vi "Variant_AppendElementToCluster.vi"(7 "Path":string, 9 "Element name":string, 10 "Element":variant, 11 "Data in":variant) -> (3 "Data out":variant)   [LabVIEW 2013, in "OpenVariant.lvlib"]
uses:
  OpenVariant.lvlib
  TypeDescriptor/OpenDescriptor.lvlib
  Conversions/OpenConvert.lvlib
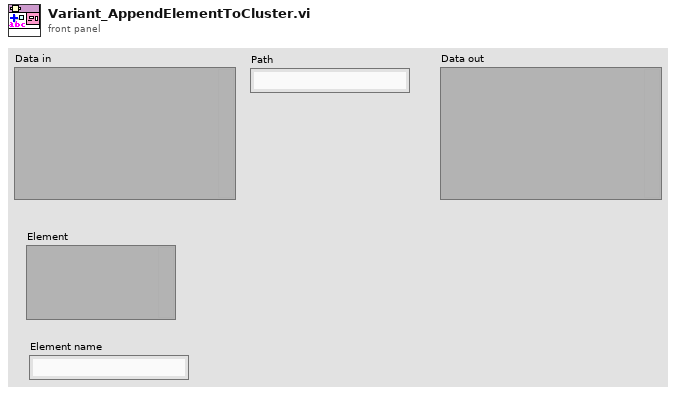
[diagram p1: front panel]
types:
  T1 = typedef "OpenDescriptor.lvlib/Descriptor Element -- cluster.ctl" = cluster{"type descriptor":i16[], "name":string, "class":string, "data string":string}
  T2 = typedef "Type Descriptor I16 Array.ctl" = T3[]
  T3 = typedef "Type Descriptor I16.ctl" = i16
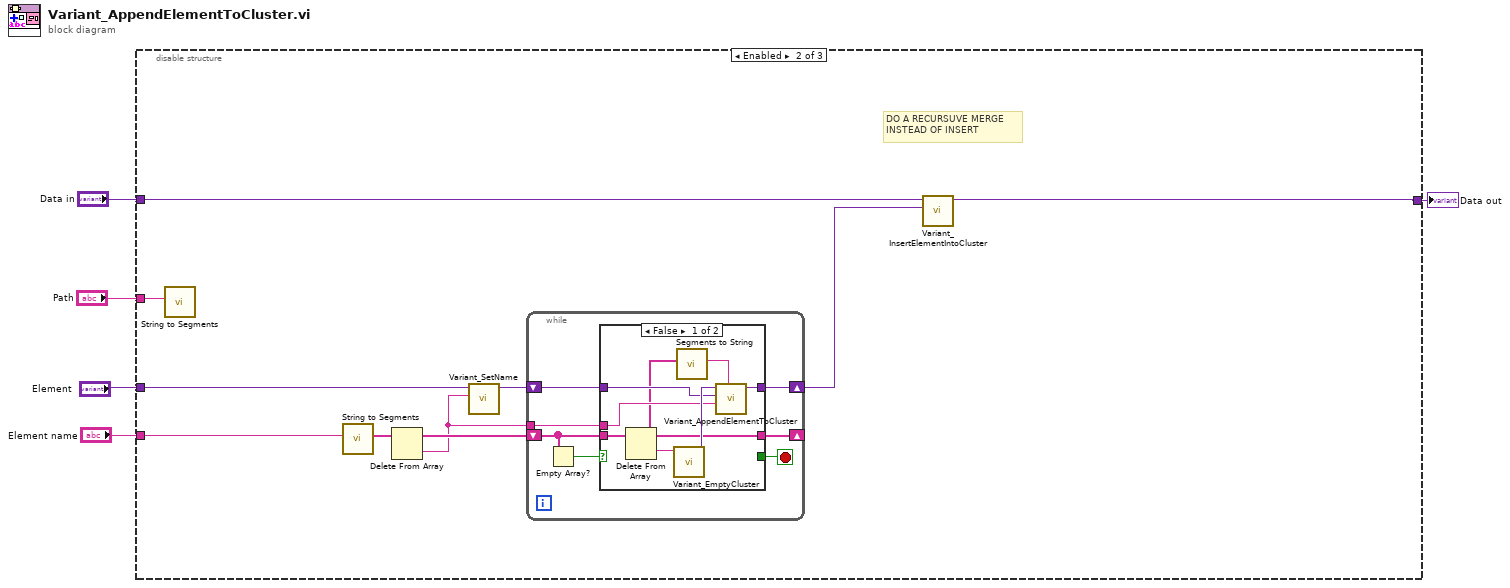
[diagram p0: block diagram]
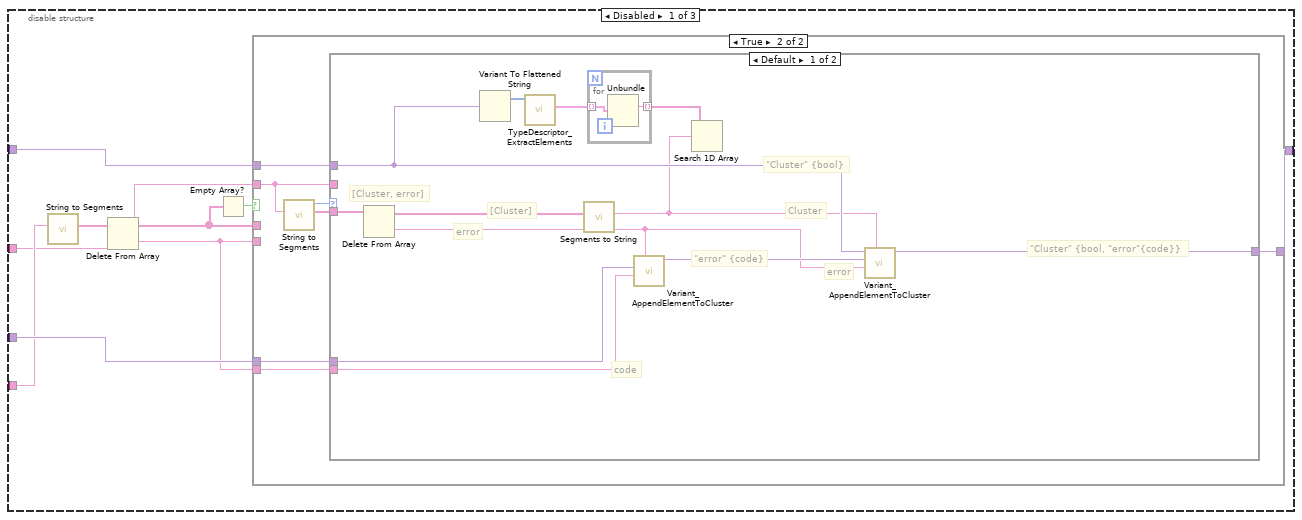
[diagram p2: hidden frame]
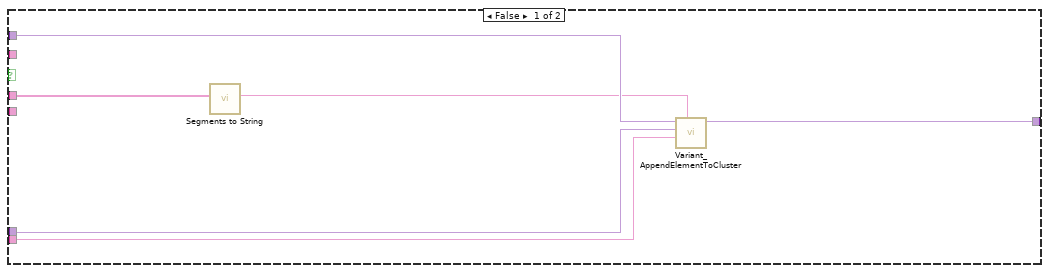
[diagram p3: hidden frame]
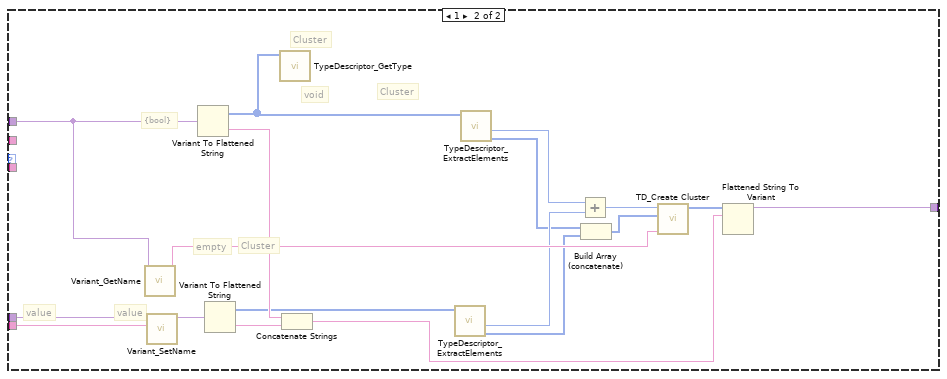
[diagram p4: hidden frame]
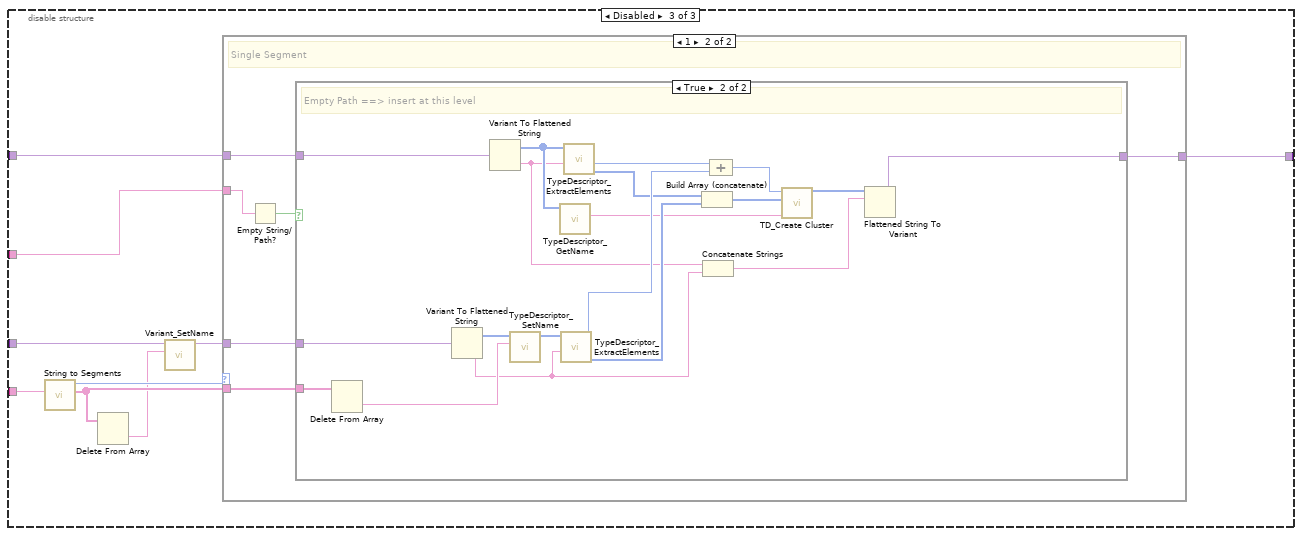
[diagram p6: hidden frame]
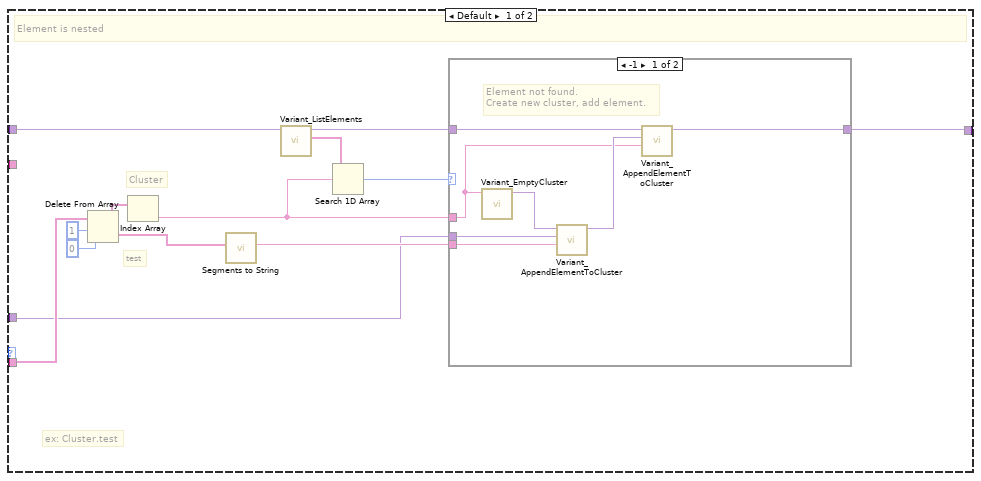
[diagram p7: hidden frame]
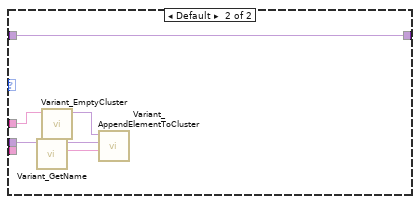
[diagram p8: hidden frame]
diagram:
  n1 = disable-structure shown="Enabled" {
    disable-tunnel: "Element" -> [w14 w67 w90]
    disable-tunnel: [w13 w62 w92] -> w4
    disable-tunnel: "Data in" -> [w12 w64 w94]
    disable-tunnel: "Element name" -> [w8 w69 w96]
    disable-tunnel: "Path" -> [w6 w60 w93]
    frame Disabled {
      n2 = call "String to Segments.vi"("String"=w8) -> ("Segments"=w11:string[])  [unwired: 9 in, 1 out]
      n3 = Delete From Array(array=w11) -> (deleted portion=w7:string, array with subset deleted=w10:string[])  [unwired: 2 in]
      n4 = Empty Array?(array=w10) -> (empty?=w9:bool)
      n5 = case shown="True" w9 {
        tunnel: w7 -> [w18 w27]
        tunnel: w14 -> [w19 w26]
        tunnel: [w20 w25] -> w13
        tunnel: w12 -> [w17 w24]
        tunnel: w7 -> [_ _]
        tunnel: w10 -> [w16 _]
        tunnel: w6 -> [_ w23]
        frame False {
          n6 = call "Segments to String.vi"("Segments"=w16) -> ("String"=w15:string)  [unwired: 10 in]
          n7 = call "Variant_AppendElementToCluster.vi"("Path"=w15, "Element name"=w18, "Element"=w19, "Data in"=w17) -> ("Data out"=w20:variant)  [unwired: 7 in]
        }
        frame True {
          n8 = call "String to Segments.vi"("String"=w23) -> ("Segments"=w21:string[], "Nb segments"=w22:i32)  [unwired: 9 in]
          n9 = case shown="Default" w22 {
            tunnel: w27 -> [w39 w57]
            tunnel: w26 -> [w38 w56]
            tunnel: [w34 w54] -> w25
            tunnel: w24 -> [w29 w52]
            tunnel: w23 -> [_ _]
            tunnel: w21 -> [w37 _]
            frame Default {
              # "\"Cluster\" {bool, \"error\"{code}}"
              # "error"
              # "\"error\" {code}"
              # "\"Cluster\" {bool}"
              # "code"
              # "error"
              # "Cluster"
              # "[Cluster]"
              # "[Cluster, error]"
              n10 = Delete From Array(array=w37) -> (deleted portion=w33:string, array with subset deleted=w36:string[])  [unwired: 2 in]
              n11 = Variant To Flattened String(Variant=w29) -> (1:w30:i16[])  [unwired: 1 out]
              n12 = call "TypeDescriptor_ExtractElements.vi"("type descriptor"=w30) -> ("elements"=w31:T1[])  [unwired: 7 in, 3 out]
              n13 = call "Segments to String.vi"("Segments"=w36) -> ("String"=w28:string)  [unwired: 10 in]
              n14 = for {
                tunnel: w31 -> [w41] mode=indexing
                tunnel: [w40] -> w32 mode=indexing
                n15 = Unbundle(w41) -> ("name"=w40:string)  [unwired: 3 out]
              }
              n16 = call "Variant_AppendElementToCluster.vi"("Path"=w33, "Element name"=w39, "Element"=w38) -> ("Data out"=w35:variant)  [unwired: 8 in]
              n17 = Search 1D Array(1D array=w32, element=w28) -> ()  [unwired: 1 in, 1 out]
              n18 = call "Variant_AppendElementToCluster.vi"("Path"=w28, "Element name"=w33, "Element"=w35, "Data in"=w29) -> ("Data out"=w34:variant)  [unwired: 7 in]
            }
            frame 1 {
              # "Cluster"
              # "Cluster"
              # "Cluster"
              # "{bool}"
              # "value"
              # "value"
              # "empty"
              # "void"
              n19 = call "Variant_GetName.vi"("Variant"=w52) -> ("Name"=w51:string)  [unwired: 8 in, 2 out]
              n20 = call "Variant_SetName.vi"("Name"=w57, "Variant"=w56) -> ("Named Variant"=w55:variant)  [unwired: 9 in]
              n21 = Variant To Flattened String(Variant=w52) -> (data string=w59:string, 1:w50:i16[])
              n22 = Variant To Flattened String(Variant=w55) -> (data string=w49:string, 1:w58:i16[])
              n23 = call "TypeDescriptor_GetType.vi"("type descriptor"=w50) -> ()  [unwired: 9 in, 2 out]
              n24 = Concatenate Strings(w59, w49) -> (w53:string)
              n25 = call "TypeDescriptor_ExtractElements.vi"("type descriptor"=w58) -> ("concatenated element descriptors"=w44:i16[], "Nb elements"=w45:i32)  [unwired: 7 in, 2 out]
              n26 = call "TypeDescriptor_ExtractElements.vi"("type descriptor"=w50) -> ("concatenated element descriptors"=w42:i16[], "Nb elements"=w43:i32)  [unwired: 7 in, 2 out]
              n27 = Add(x=w43, y=w45) -> (x+y=w46:i32)
              n28 = Build Array (concatenate)(w42, w44) -> (w48:i16[])
              n29 = call <vilib>:"TD_Create Cluster.vi"("Name"=w51, "Concatenated Elts"=w48, "N Elts"=w46) -> ("ClusterTD"=w47:T2)  [unwired: 8 in]
              n30 = Flattened String To Variant(6:w53, 7:w47) -> (3:w54:variant)  [unwired: 1 in, 1 out]
            }
          }
        }
      }
    }
    frame Enabled {
      # "DO A RECURSUVE MERGE\nINSTEAD OF INSERT"
      n31 = call "String to Segments.vi"("String"=w60) -> ()  [unwired: 9 in, 2 out]
      n32 = call "String to Segments.vi"("String"=w69) -> ("Segments"=w68:string[])  [unwired: 9 in, 1 out]
      n33 = Delete From Array(array=w68) -> (deleted portion=w61:string, array with subset deleted=w66:string[])  [unwired: 2 in]
      n34 = call "Variant_SetName.vi"("Name"=w61, "Variant"=w67) -> ("Named Variant"=w65:variant)  [unwired: 9 in]
      n35 = while {
        shift-right: [w74] -> _
        shift-left: w66 -> [w73]
        shift-right: [w71] -> w63
        shift-left: w65 -> [w72]
        tunnel: w61 -> [w70]
        stop <- w75 stop-if-true
        n36 = Empty Array?(array=w73) -> (empty?=w76:bool)
        n37 = case shown="False" w76 {
          selector: w76 -> [_ w87]
          tunnel: [_ w87] -> w75
          tunnel: [w78 w86] -> w74
          tunnel: w73 -> [w84 w86]
          tunnel: w72 -> [w82 w85]
          tunnel: [w81 w85] -> w71
          tunnel: w70 -> [w79 _]
          frame False {
            n38 = Delete From Array(array=w84) -> (deleted portion=w80:string, array with subset deleted=w78:string[])  [unwired: 2 in]
            n39 = call "Variant_EmptyCluster.vi"("Cluster Name"=w80) -> ("Empty Cluster"=w83:variant)  [unwired: 10 in]
            n40 = call "Segments to String.vi"("Segments"=w78) -> ("String"=w77:string)  [unwired: 10 in]
            n41 = call "Variant_AppendElementToCluster.vi"("Path"=w77, "Element name"=w79, "Element"=w82, "Data in"=w83) -> ("Data out"=w81:variant)  [unwired: 7 in]
          }
          frame True {
          }
        }
      }
      n42 = call "Variant_InsertElementIntoCluster.vi"("Element"=w63, "Cluster in"=w64) -> ("Cluster out"=w62:variant)  [unwired: 9 in]
    }
    frame Disabled {
      n43 = call "String to Segments.vi"("String"=w96) -> ("Segments"=w91:string[], "Nb segments"=w95:i32)  [unwired: 9 in]
      n44 = Delete From Array(array=w91) -> (deleted portion=w88:string)  [unwired: 2 in, 1 out]
      n45 = call "Variant_SetName.vi"("Name"=w88, "Variant"=w90) -> ("Named Variant"=w89:variant)  [unwired: 9 in]
      n46 = case shown="1" w95 {
        tunnel: w94 -> [w102 w128]
        tunnel: w93 -> [_ w127]
        tunnel: w89 -> [w103 w125]
        tunnel: [w97 w124] -> w92
        tunnel: w91 -> [w109 w123]
        frame Default {
          # "test"
          # "Cluster"
          # "ex: Cluster.test"
          # "Element is nested"
          n47 = Delete From Array(array=w109, length=1, index=0) -> (deleted portion=w105:string[], array with subset deleted=w106:string[])
          n48 = Index Array(array=w106) -> (element=w100:string)  [unwired: 1 in]
          n49 = call "Segments to String.vi"("Segments"=w105) -> ("String"=w104:string)  [unwired: 10 in]
          n50 = call "Variant_ListElements.vi"("Variant"=w102) -> ("element names"=w101:string[], "Variant dup"=w98:variant)  [unwired: 7 in, 2 out]
          n51 = Search 1D Array(1D array=w101, element=w100) -> (index of element=w99:i32)  [unwired: 1 in]
          n52 = case shown="-1" w99 {
            tunnel: w104 -> [w114 _]
            tunnel: w103 -> [w115 w119]
            tunnel: w100 -> [w111 w121]
            tunnel: w98 -> [w113 w117]
            tunnel: [w110 w117] -> w97
            frame -1 {
              # "Element not found.\nCreate new cluster, add element."
              n53 = call "Variant_EmptyCluster.vi"("Cluster Name"=w111) -> ("Empty Cluster"=w116:variant)  [unwired: 10 in]
              n54 = call "Variant_AppendElementToCluster.vi"("Element name"=w114, "Element"=w115, "Data in"=w116) -> ("Data out"=w112:variant)  [unwired: 8 in]
              n55 = call "Variant_AppendElementToCluster.vi"("Element name"=w111, "Element"=w112, "Data in"=w113) -> ("Data out"=w110:variant)  [unwired: 8 in]
            }
            frame Default {
              n56 = call "Variant_GetName.vi"("Variant"=w119) -> ("Name"=w120:string, "Variant dup"=w118:variant)  [unwired: 8 in, 1 out]
              n57 = call "Variant_EmptyCluster.vi"("Cluster Name"=w121) -> ("Empty Cluster"=w122:variant)  [unwired: 10 in]
              n58 = call "Variant_AppendElementToCluster.vi"("Element name"=w120, "Element"=w118, "Data in"=w122) -> ()  [unwired: 8 in, 1 out]
            }
          }
        }
        frame 1 {
          # "Single Segment"
          n59 = Empty String/Path?(string/path=w127) -> (empty?=w126:bool)
          n60 = case shown="True" w126 {
            tunnel: w128 -> [w129 w148]
            tunnel: w125 -> [_ w135]
            tunnel: [w129 w139] -> w124
            tunnel: w123 -> [_ w136]
            frame False {
            }
            frame True {
              # "Empty Path ==> insert at this level"
              n61 = Delete From Array(array=w136) -> (deleted portion=w132:string)  [unwired: 2 in, 1 out]
              n62 = Variant To Flattened String(Variant=w135) -> (data string=w131:string, 1:w134:i16[])
              n63 = Variant To Flattened String(Variant=w148) -> (data string=w130:string, 1:w138:i16[])
              n64 = call "TypeDescriptor_SetName.vi"("name"=w132, "type descriptor"=w134) -> ("type descriptor dup"=w133:i16[])  [unwired: 7 in, 2 out]
              n65 = call "TypeDescriptor_GetName.vi"("type descriptor"=w138) -> ("name"=w137:string)  [unwired: 8 in, 2 out]
              n66 = call "TypeDescriptor_ExtractElements.vi"("Data String"=w131, "type descriptor"=w133) -> ("concatenated element descriptors"=w144:i16[], "Nb elements"=w146:i32)  [unwired: 6 in, 2 out]
              n67 = call "TypeDescriptor_ExtractElements.vi"("Data String"=w130, "type descriptor"=w138) -> ("concatenated element descriptors"=w145:i16[], "Nb elements"=w147:i32)  [unwired: 6 in, 2 out]
              n68 = Build Array (concatenate)(w145, w144) -> (w141:i16[])
              n69 = Concatenate Strings(w130, w131) -> (w140:string)
              n70 = Compound Arithmetic op=ADD(w147, w146) -> (w142:i32)
              n71 = call <vilib>:"TD_Create Cluster.vi"("Name"=w137, "Concatenated Elts"=w141, "N Elts"=w142) -> ("ClusterTD"=w143:T2)  [unwired: 8 in]
              n72 = Flattened String To Variant(6:w140, 7:w143) -> (3:w139:variant)  [unwired: 1 in, 1 out]
            }
          }
        }
      }
    }
  }
  "Data out" <- w4
